vi "SLSC-12201 Enable_Disable Channel.vi"(7 "Item Ref in":T1 format="%.0x", 8 "error in (no error)":errorcluster, 9 "Enable":bool, 10 "Tree":string[](array[string]), 11 "TreeControl in":refnum<vi>) -> (0 "error out":errorcluster, 3 "Boolean":bool)   [LabVIEW 2020, in "SLSC-12201 DIO System Explorer.lvlib"]
uses:
  SLSC-12201 DIO System Explorer.lvlib
  <vilib>/NI VeriStand/Custom Device API/Custom Device Item Ref.ctl
  <vilib>/NI VeriStand/Custom Device Tools/Custom Device Utility Library/NI VeriStand - Search for Item by Name.vi
  <vilib>/NI VeriStand/Custom Device Tools/Custom Device Utility Library/Custom Device Utility Library.lvlib
  <vilib>/NI VeriStand/Custom Device API/Custom Device API.lvlib
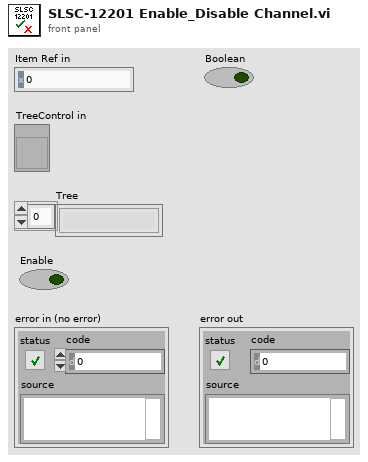
[diagram p1: front panel]
types:
  T1 = typedef "Custom Device API.lvlib/Custom Device Item Ref.ctl" = u64
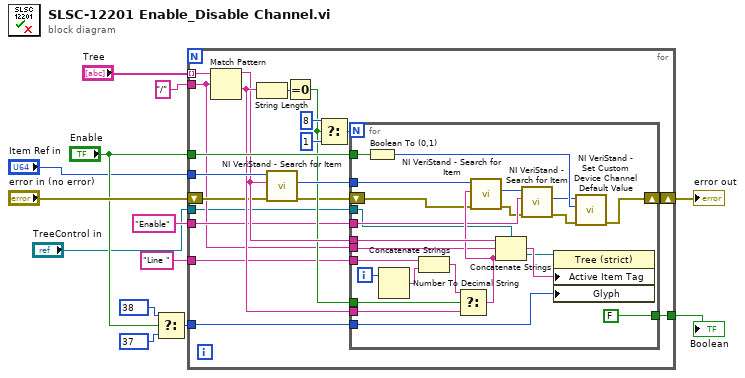
[diagram p0: block diagram]
diagram:
  n1 = Select(t=38, s="Enable", f=37) -> (s? t:f=w7:i32)
  n2 = for {
    tunnel: "Tree" -> [w27] mode=indexing
    tunnel: w7 -> [w29]
    tunnel: "Item Ref in" -> [w28]
    tunnel: "Enable" -> [w25]
    tunnel: [w23] -> w8
    tunnel: "/" ("regular expression") -> [w15]
    tunnel: "Line " ("string") -> [w20]
    tunnel: "Enable" ("Item Name") -> [w19]
    shift-right: [w16] -> w13
    shift-left: "error in (no error)" -> [w18]
    tunnel: "TreeControl in" -> [w14]
    n3 = Match Pattern(string=w27, regular expression=w15) -> (before substring=w22:string, after substring=w24:string)  [unwired: 1 in, 2 out]
    n4 = String Length(string=w24) -> (length=w33:i32)
    n5 = call-poly <vilib>:"NI VeriStand - Search for Item.vi"("error in"=w18, "Item Name"=w22, "Section Ref in"=w28) -> ("error out"=w17:errorcluster, "Item Ref"=w26:T1)  [unwired: 5 in, 2 out]
    n6 = Equal To 0?(x=w33) -> (x = 0?=w21:bool)
    n7 = Select(t=8, s=w21, f=1) -> (s? t:f=w32:i32)
    n8 = for {
      N: w32 -> [_]
      tunnel: w22 -> [w52]
      tunnel: w29 -> [w54]
      tunnel: w26 -> [w53]
      tunnel: w25 -> [w50]
      tunnel: w21 -> [w46]
      tunnel: w24 -> [w43]
      tunnel: [FALSE] -> w23
      tunnel: w20 -> [w41]
      tunnel: w19 -> [w40]
      shift-right: [w36] -> w16
      shift-left: w17 -> [w39]
      tunnel: w15 -> [w35]
      tunnel: w14 -> [w34]
      i -> [w56]
      n9 = Boolean To (0,1)(Boolean=w50) -> (0, 1=w49:i16)
      n10 = Number To Decimal String(number=w56) -> (decimal integer string=w55:string)  [unwired: 1 in]
      n11 = Concatenate Strings(w41, w55) -> (w45:string)
      n12 = Select(t=w45, s=w46, f=w43) -> (s? t:f=w44:string)
      n13 = call-poly <vilib>:"NI VeriStand - Search for Item.vi"("error in"=w39, "Item Name"=w44, "Section Ref in"=w53) -> ("error out"=w38:errorcluster, "Item Ref"=w48:T1)  [unwired: 5 in, 2 out]
      n14 = Concatenate Strings(w52, w35, w44) -> (w51:string)
      n15 = call-poly <vilib>:"NI VeriStand - Search for Item.vi"("error in"=w38, "Item Name"=w40, "Section Ref in"=w48) -> ("error out"=w37:errorcluster, "Item Ref"=w47:T1)  [unwired: 5 in, 2 out]
      n16 = property on="Property Node" class="Tree (strict)"(reference=w34, "Active Item Tag"=w51, "Glyph"=w54) -> ()  [unwired: 1 in, 2 out]
      n17 = call <vilib>:"NI VeriStand - Set Custom Device Channel Default Value.vi"("error in (no error)"=w37, "Default Value"=w49, "Channel Ref in"=w47) -> ("error out"=w36:errorcluster)  [unwired: 7 in, 1 out]
    }
  }
  "error out" <- w13
  "Boolean" <- w8
